vi "Init.vi"(8 "error in":errorcluster, 10 "<JSON> Const Action Data":string, 11 "Perform Action HSU MCU Read Strategy in":refnum<class "Perform Action HSU MCU Strategy.lvclass">) -> (0 "error out":errorcluster, 3 "Perform Action HSU MCU Read Strategy out":refnum<class "Perform Action HSU MCU Strategy.lvclass">)   [LabVIEW 2023, in "Perform Action HSU MCU Strategy.lvclass"]
uses:
  Perform Action HSU MCU Strategy.lvclass
  Perform Action HSU MCU Strategy.lvclass/Perform Action HSU MCU Strategy.ctl
  a7101a50-3e58-4459-95a3-d8610910b48d.vi
  <vilib>/JDP Science/JSONtext/JSON text to Variant.vi
  <vilib>/JDP Science/JSONtext/LVClass Serializer/JSONtext LVClass Serializer.lvclass
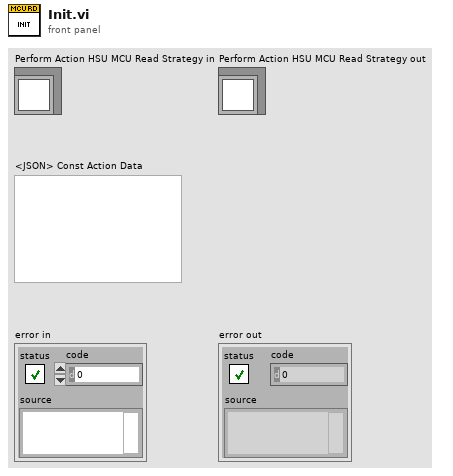
[diagram p1: front panel]
types:
  T1 = cluster{"Action":enum16{"Read", "Write"}, "MCU":string, "Attribute":string, "Value":variant}
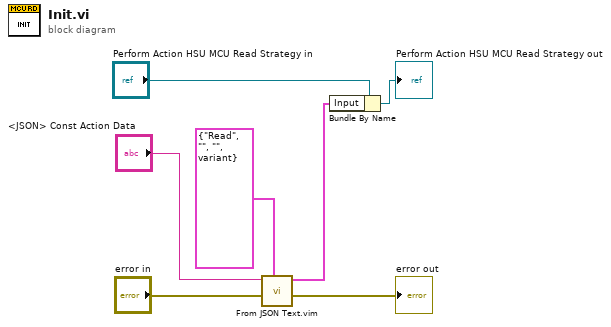
[diagram p0: block diagram]
diagram:
  n1 = call "From JSON Text.vim"("Data Type and Default Value"=T1 {"Action"=enum."Read", "MCU"="", "Attribute"="", "Value"=variant}, "error in (no error)"="error in", "JSON"="<JSON> Const Action Data") -> ("error out"=→"error out":errorcluster, "Data out"=w1:T1)  [unwired: 7 in]
  n2 = Bundle By Name(cluster="Perform Action HSU MCU Read Strategy in", "Input"=w1) -> (→"Perform Action HSU MCU Read Strategy out":refnum<class "Perform Action HSU MCU Strategy.lvclass">)
